vi "READ SG AND T VALUE.vi"(11 "Mod 1":T1) -> (3 "Array":string[](array[string]))   [LabVIEW 2019]
uses:
  BenchSelector.vi
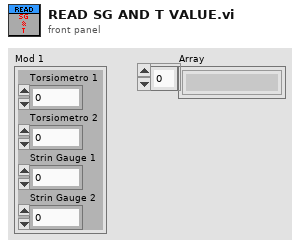
[diagram p1: front panel]
types:
  T1 = cluster{"Torsiometro 1":dbl, "Torsiometro 2":dbl, "Strin Gauge 1":dbl, "Strin Gauge 2":dbl}
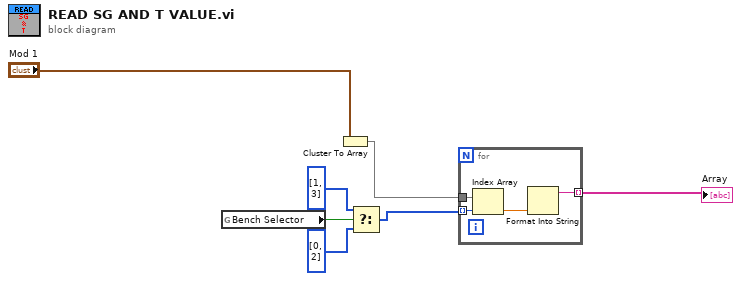
[diagram p0: block diagram]
diagram:
  n1 = global read "BenchSelector.vi" "Bench Selector"() -> (w4:bool)
  n2 = Cluster To Array(cluster="Mod 1") -> (array=w5:dbl[])
  n3 = Select(t=i32[] [1, 3], s=w4, f=i32[] [0, 2]) -> (s? t:f=w6:i32[])
  n4 = for {
    tunnel: w5 -> [w11]
    tunnel: w6 -> [w10] mode=indexing
    tunnel: [w8] -> w7 mode=indexing
    n5 = Index Array(array=w11, index=w10) -> (element=w9:dbl)
    n6 = Format Into String(w9) -> (resulting string=w8:string)  [unwired: 3 in, 1 out]
  }
  "Array" <- w7
